vi "Firmware Filename Parser.vi"(0 "filename":string, 7 "firmware name":string, 11 "current versions":u8[](array[numeric])) -> (8 "update firmware":bool)   [LabVIEW 2010]
panel:
  out "assembly v (file)":dbl
  out "hw v (file)":dbl
  out "harp v (file)":dbl
  out "fw v (file)":dbl
  out "hw v (current)":dbl
  out "ass v (current)":dbl
  out "harp v (current)":dbl
  out "fw v (current)":dbl
  out "fw v":string
  out "harp v":string
  out "hw v":string
  out "assembly v":string
  out "assembly":string
  out "hw":string
  out "harp":string
  out "fw":string
  # "Delete this labels (debug only):"
  # "LedArray-fw2.2-harp1.4-hw1.x-ass0.hex"
  # "LedArray-fw2.2-harp1.4-hw1.3-ass0.hex"
  # "Behavior-fw2.2-harp1.4-hw1.0-ass2.hex"
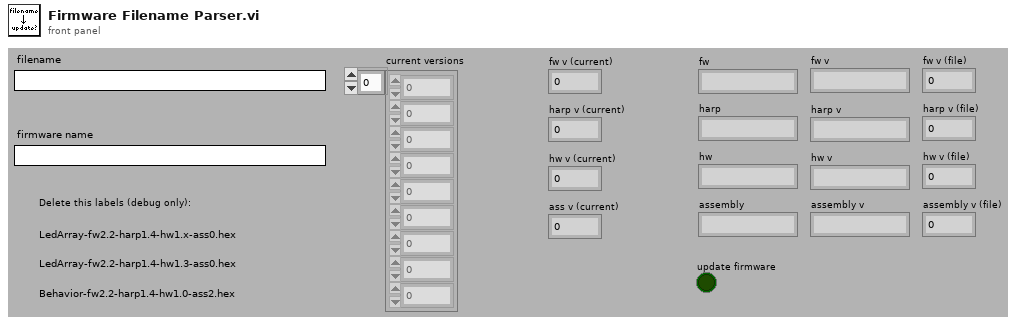
[diagram p1: front panel]
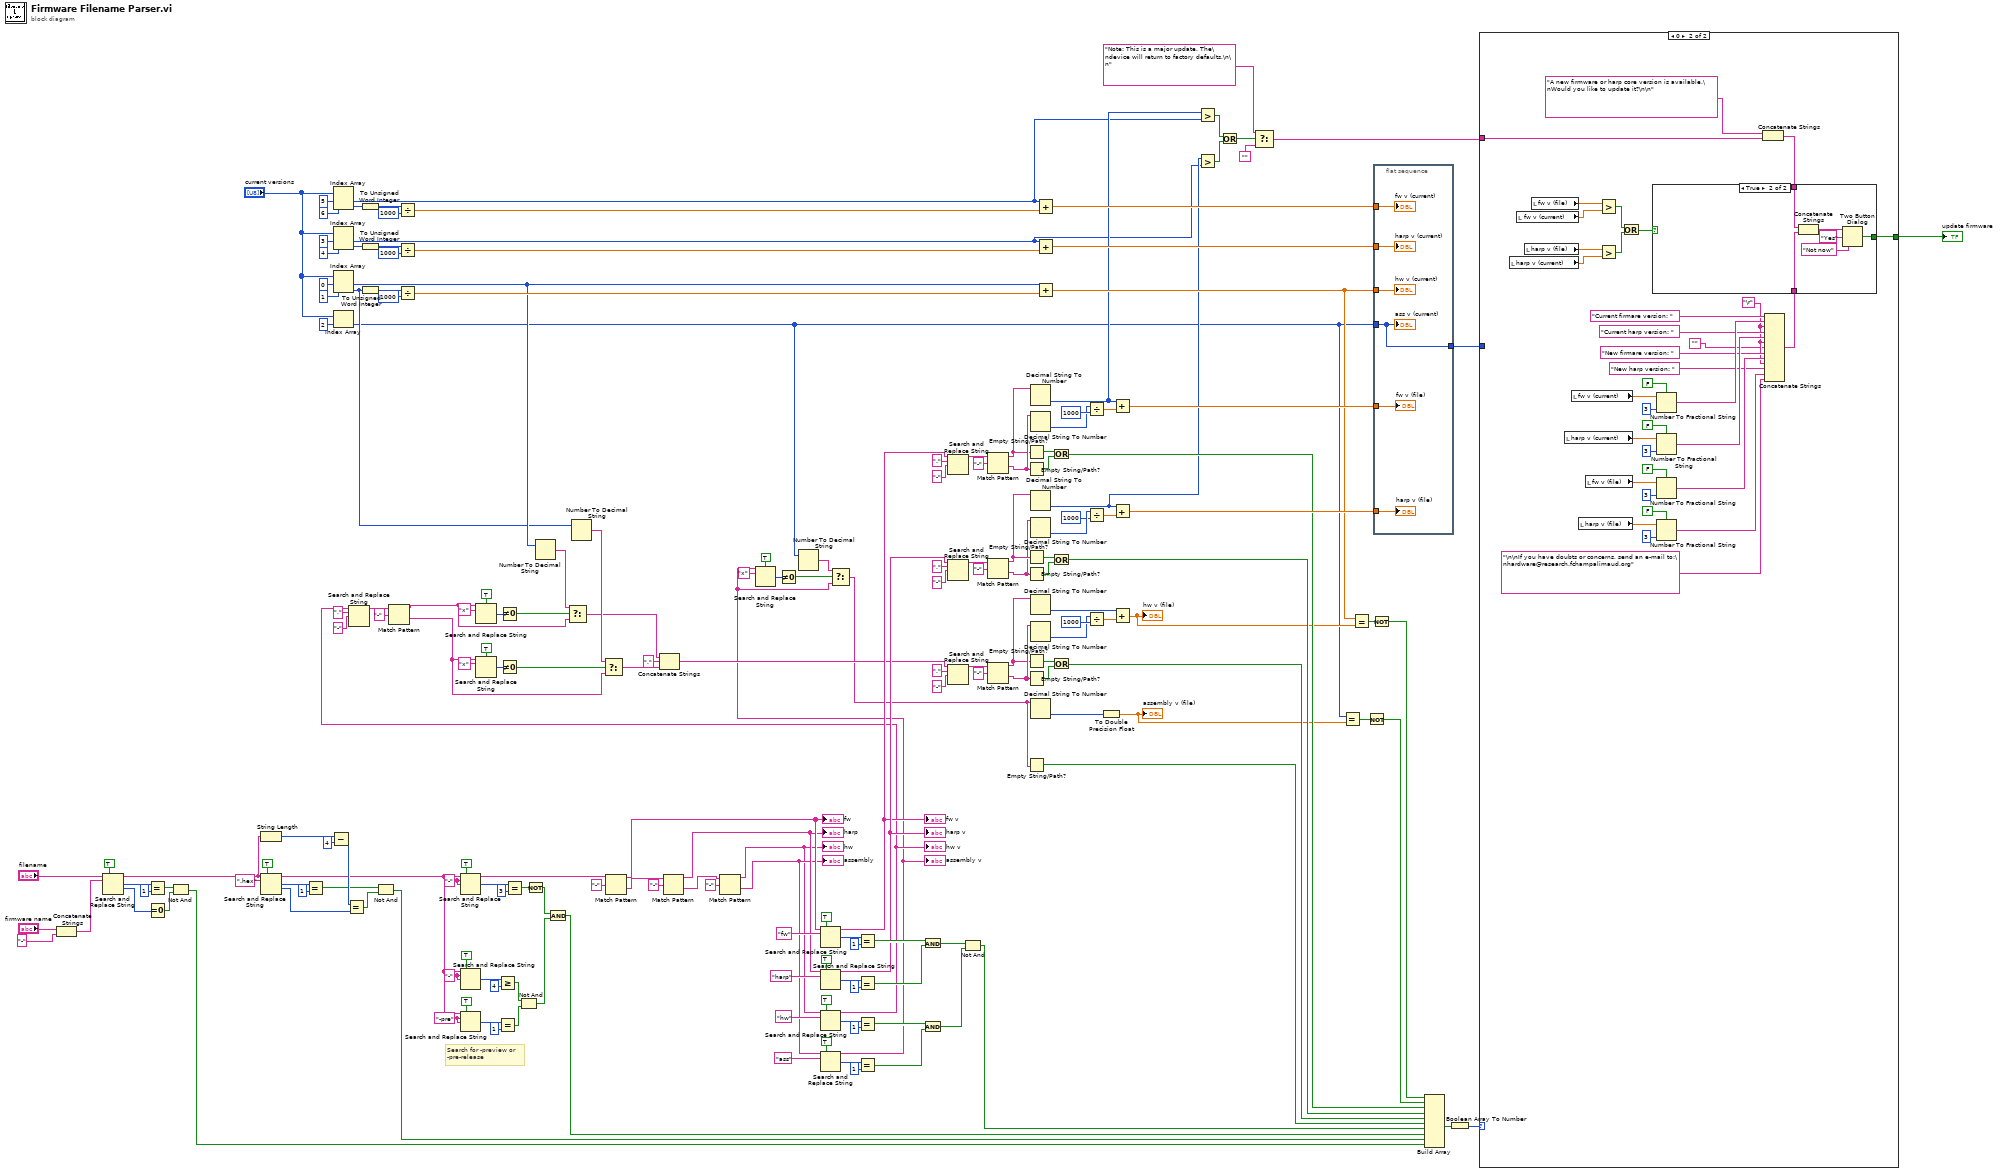
[diagram p0: block diagram]
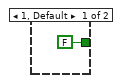
[diagram p2: hidden frame]
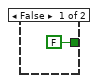
[diagram p3: hidden frame]
diagram:
  w7 = "-pre" ("search string")
  w12 = "-" ("search string")
  w170 = "-" ("search string")
  # "Search for -preview or\n-pre-release"
  n1 = Concatenate Strings("firmware name", "-" ("string")) -> (w188:string)
  n2 = Search and Replace String(replace all?=TRUE ("replace all? (F)"), input string="filename", search string=w188) -> (result string=w180:string, number of replacements=w187:i32, offset past replacement=w186:i32)  [unwired: 5 in, 1 out]
  n3 = Equal?(x=w187, y=1) -> (x = y?=w183:bool)
  n4 = Equal To 0?(x=w186) -> (x = 0?=w184:bool)
  n5 = Not And(1:w184, 2:w183) -> (0:w167:bool)
  n6 = String Length(string=w180) -> (length=w178:i32)
  n7 = Search and Replace String(replace all?=TRUE ("replace all? (F)"), input string=w180, search string=".hex") -> (result string=w5:string, number of replacements=w182:i32, offset past replacement=w175:i32)  [unwired: 5 in, 1 out]
  n8 = Equal?(x=w182, y=1) -> (x = y?=w173:bool)
  n9 = Subtract(x=w178, y=4) -> (x-y=w176:i32)
  n10 = Index Array(array="current versions", index #1=5 ("index"), index #2=6 ("index")) -> (element #1=w52:u8, element #2=w129:u8)
  n11 = Index Array(array="current versions", index #1=3 ("index"), index #2=4 ("index")) -> (element #1=w50:u8, element #2=w120:u8)
  n12 = Index Array(array="current versions", index #1=0 ("index"), index #2=1 ("index")) -> (element #1=w37:u8, element #2=w34:u8)
  n13 = Index Array(array="current versions", index=2) -> (element=w14:u8)
  n14 = Equal?(x=w176, y=w175) -> (x = y?=w174:bool)
  n15 = To Unsigned Word Integer(number=w129) -> (unsigned 16bit integer=w127:u16)
  n16 = To Unsigned Word Integer(number=w120) -> (unsigned 16bit integer=w122:u16)
  n17 = To Unsigned Word Integer(number=w34) -> (unsigned 16bit integer=w115:u16)
  n18 = Not And(1:w174, 2:w173) -> (0:w168:bool)
  n19 = Divide(x=w127, y=u16 1000) -> (x/y=w126:dbl)
  n20 = Divide(x=w122, y=u16 1000) -> (x/y=w123:dbl)
  n21 = Divide(x=w115, y=u16 1000) -> (x/y=w116:dbl)
  n22 = Search and Replace String(replace all?=TRUE ("replace all? (F)"), input string=w5, search string=w170, replace string=w170) -> (result string=w163:string, number of replacements=w171:i32)  [unwired: 4 in, 2 out]
  n23 = Search and Replace String(replace all?=TRUE ("replace all? (F)"), input string=w5, search string=w12, replace string=w12) -> (number of replacements=w11:i32)  [unwired: 4 in, 3 out]
  n24 = Search and Replace String(replace all?=TRUE ("replace all? (F)"), input string=w5, search string=w7, replace string=w7) -> (number of replacements=w8:i32)  [unwired: 4 in, 3 out]
  n25 = Greater Or Equal?(x=w11, y=4) -> (x >= y?=w3:bool)
  n26 = Equal?(x=w8, y=1) -> (x = y?=w4:bool)
  n27 = Equal?(x=w171, y=3) -> (x = y?=w169:bool)
  n28 = Not And(1:w4, 2:w3) -> (0:w1:bool)
  n29 = Not(x=w169) -> (.not. x?=w105:bool)
  n30 = Number To Decimal String(number=w37) -> (decimal integer string=w36:string)  [unwired: 1 in]
  n31 = And(x=w105, y=w1) -> (x .and. y?=w2:bool)
  n32 = Number To Decimal String(number=w34) -> (decimal integer string=w35:string)  [unwired: 1 in]
  n33 = Match Pattern(string=w163, regular expression="-") -> (before substring=w141:string, after substring=w160:string)  [unwired: 1 in, 2 out]
  "fw" <- w141
  n34 = Match Pattern(string=w160, regular expression="-") -> (before substring=w140:string, after substring=w158:string)  [unwired: 1 in, 2 out]
  "harp" <- w140
  n35 = Match Pattern(string=w158, regular expression="-") -> (before substring=w39:string, after substring=w139:string)  [unwired: 1 in, 2 out]
  "hw" <- w39
  "assembly" <- w139
  n36 = Number To Decimal String(number=w14) -> (decimal integer string=w17:string)  [unwired: 1 in]
  n37 = Search and Replace String(replace all?=TRUE ("replace all? (F)"), input string=w141, search string="fw") -> (result string=w72:string, number of replacements=w155:i32)  [unwired: 5 in, 2 out]
  "fw v" <- w72
  n38 = Search and Replace String(replace all?=TRUE ("replace all? (F)"), input string=w140, search string="harp") -> (result string=w73:string, number of replacements=w152:i32)  [unwired: 5 in, 2 out]
  "harp v" <- w73
  n39 = Search and Replace String(replace all?=TRUE ("replace all? (F)"), input string=w39, search string="hw") -> (result string=w26:string, number of replacements=w147:i32)  [unwired: 5 in, 2 out]
  "hw v" <- w26
  n40 = Search and Replace String(input string=w26, search string=".", replace string="-" ("replace string (\"\")")) -> (result string=w25:string)  [unwired: 5 in, 3 out]
  n41 = Match Pattern(string=w25, regular expression="-") -> (before substring=w24:string, after substring=w23:string)  [unwired: 1 in, 2 out]
  n42 = Search and Replace String(case sensitive?=TRUE ("ignore case? (F)"), input string=w24, search string="x") -> (number of replacements=w43:i32)  [unwired: 5 in, 3 out]
  n43 = Search and Replace String(case sensitive?=TRUE ("ignore case? (F)"), input string=w23, search string="x") -> (number of replacements=w42:i32)  [unwired: 5 in, 3 out]
  n44 = Not Equal To 0?(x=w43) -> (x != 0?=w38:bool)
  n45 = Not Equal To 0?(x=w42) -> (x != 0?=w30:bool)
  n46 = Select(t=w36, s=w38, f=w24) -> (s? t:f=w33:string)
  n47 = Select(t=w35, s=w30, f=w23) -> (s? t:f=w32:string)
  n48 = Concatenate Strings(w33, "." ("string"), w32) -> (w22:string)
  n49 = Search and Replace String(replace all?=TRUE ("replace all? (F)"), input string=w139, search string="ass") -> (result string=w16:string, number of replacements=w144:i32)  [unwired: 5 in, 2 out]
  "assembly v" <- w16
  n50 = Search and Replace String(case sensitive?=TRUE ("ignore case? (F)"), input string=w16, search string="x") -> (number of replacements=w19:i32)  [unwired: 5 in, 3 out]
  n51 = Not Equal To 0?(x=w19) -> (x != 0?=w18:bool)
  n52 = Select(t=w17, s=w18, f=w16) -> (s? t:f=w15:string)
  n53 = Equal?(x=w155, y=1) -> (x = y?=w138:bool)
  n54 = Equal?(x=w152, y=1) -> (x = y?=w137:bool)
  n55 = Equal?(x=w147, y=1) -> (x = y?=w136:bool)
  n56 = Equal?(x=w144, y=1) -> (x = y?=w135:bool)
  n57 = And(x=w138, y=w137) -> (x .and. y?=w134:bool)
  n58 = And(x=w136, y=w135) -> (x .and. y?=w133:bool)
  n59 = Search and Replace String(input string=w72, search string=".", replace string="-" ("replace string (\"\")")) -> (result string=w100:string)  [unwired: 5 in, 3 out]
  n60 = Search and Replace String(input string=w73, search string=".", replace string="-" ("replace string (\"\")")) -> (result string=w95:string)  [unwired: 5 in, 3 out]
  n61 = Search and Replace String(input string=w22, search string=".", replace string="-" ("replace string (\"\")")) -> (result string=w76:string)  [unwired: 5 in, 3 out]
  n62 = Not And(1:w133, 2:w134) -> (0:w132:bool)
  n63 = Match Pattern(string=w100, regular expression="-") -> (before substring=w106:string, after substring=w107:string)  [unwired: 1 in, 2 out]
  n64 = Match Pattern(string=w95, regular expression="-") -> (before substring=w90:string, after substring=w89:string)  [unwired: 1 in, 2 out]
  n65 = Match Pattern(string=w76, regular expression="-") -> (before substring=w81:string, after substring=w82:string)  [unwired: 1 in, 2 out]
  n66 = Empty String/Path?(string/path=w106) -> (empty?=w108:bool)
  n67 = Empty String/Path?(string/path=w107) -> (empty?=w109:bool)
  n68 = Empty String/Path?(string/path=w90) -> (empty?=w88:bool)
  n69 = Empty String/Path?(string/path=w89) -> (empty?=w87:bool)
  n70 = Empty String/Path?(string/path=w81) -> (empty?=w83:bool)
  n71 = Empty String/Path?(string/path=w82) -> (empty?=w84:bool)
  n72 = Empty String/Path?(string/path=w15) -> (empty?=w68:bool)
  n73 = Decimal String To Number(string=w106) -> (number=w53:i32)  [unwired: 2 in, 1 out]
  n74 = Decimal String To Number(string=w107) -> (number=w101:i32)  [unwired: 2 in, 1 out]
  n75 = Decimal String To Number(string=w90) -> (number=w51:i32)  [unwired: 2 in, 1 out]
  n76 = Decimal String To Number(string=w89) -> (number=w94:i32)  [unwired: 2 in, 1 out]
  n77 = Decimal String To Number(string=w81) -> (number=w78:i32)  [unwired: 2 in, 1 out]
  n78 = Decimal String To Number(string=w82) -> (number=w77:i32)  [unwired: 2 in, 1 out]
  n79 = Decimal String To Number(string=w15) -> (number=w66:i32)  [unwired: 2 in, 1 out]
  n80 = Add(x=w52, y=w126) -> (x+y=w125:dbl)
  n81 = Add(x=w50, y=w123) -> (x+y=w124:dbl)
  n82 = Add(x=w37, y=w116) -> (x+y=w63:dbl)
  n83 = Or(x=w108, y=w109) -> (x .or. y?=w71:bool)
  n84 = Or(x=w88, y=w87) -> (x .or. y?=w70:bool)
  n85 = Or(x=w83, y=w84) -> (x .or. y?=w69:bool)
  n86 = Divide(x=w101, y=u16 1000) -> (x/y=w103:dbl)
  n87 = Divide(x=w94, y=u16 1000) -> (x/y=w92:dbl)
  n88 = Divide(x=w77, y=u16 1000) -> (x/y=w79:dbl)
  n89 = To Double Precision Float(number=w66) -> (double precision float=w65:dbl)
  "assembly v (file)" <- w65
  n90 = Add(x=w53, y=w103) -> (x+y=w102:dbl)
  n91 = Add(x=w51, y=w92) -> (x+y=w93:dbl)
  n92 = Add(x=w78, y=w79) -> (x+y=w64:dbl)
  "hw v (file)" <- w64
  n93 = Greater?(x=w53, y=w52) -> (0:w55:bool)
  n94 = Greater?(x=w51, y=w50) -> (0:w54:bool)
  n95 = Or(x=w55, y=w54) -> (x .or. y?=w49:bool)
  n96 = Select(t="Note: This is a major update. The\ndevice will return to factory defaults.\n\n" ("message"), s=w49, f="") -> (s? t:f=w46:string)
  n97 = Equal?(x=w14, y=w65) -> (x = y?=w61:bool)
  n98 = Equal?(x=w63, y=w64) -> (x = y?=w62:bool)
  n99 = Not(x=w61) -> (.not. x?=w60:bool)
  n100 = Not(x=w62) -> (.not. x?=w59:bool)
  n101 = flat-sequence {
    tunnel: w125 -> [w197]
    tunnel: w124 -> [w196]
    tunnel: w102 -> [w195]
    tunnel: w93 -> [w194]
    tunnel: w14 -> [w192]
    tunnel: w63 -> [w193]
    tunnel: [w192] -> w57
    frame #0 {
      "fw v (current)" <- w197
      "harp v (current)" <- w196
      "hw v (current)" <- w193
      "ass v (current)" <- w192
      "fw v (file)" <- w195
      "harp v (file)" <- w194
    }
  }
  n102 = Build Array(w59, w60, w71, w70, w69, w68, w132, w2, w168, w167) -> (w67:bool[])
  n103 = Boolean Array To Number(Boolean array=w67) -> (number=w58:u32)
  n104 = case shown="0" w58 {
    tunnel: w57 -> [_ _]
    tunnel: [FALSE ("T button?") w206] -> w56
    tunnel: w46 -> [_ w202]
    frame 1, Default {
    }
    frame 0 {
      w211 = "\r"
      n105 = local read "harp v (current)"() -> (w231:dbl)
      n106 = local read "fw v (current)"() -> (w232:dbl)
      n107 = local read "harp v (file)"() -> (w230:dbl)
      n108 = local read "fw v (file)"() -> (w233:dbl)
      n109 = local read "harp v (current)"() -> (w222:dbl)
      n110 = local read "fw v (current)"() -> (w225:dbl)
      n111 = local read "harp v (file)"() -> (w221:dbl)
      n112 = local read "fw v (file)"() -> (w218:dbl)
      n113 = Greater?(x=w233, y=w232) -> (0:w228:bool)
      n114 = Greater?(x=w230, y=w231) -> (0:w229:bool)
      n115 = Or(x=w228, y=w229) -> (x .or. y?=w207:bool)
      n116 = Number To Fractional String(use system decimal point (T)=FALSE, number=w225, precision (6)=i16 3) -> (F-format string=w216:string)  [unwired: 1 in]
      n117 = Number To Fractional String(use system decimal point (T)=FALSE, number=w222, precision (6)=i16 3) -> (F-format string=w214:string)  [unwired: 1 in]
      n118 = Number To Fractional String(use system decimal point (T)=FALSE, number=w218, precision (6)=i16 3) -> (F-format string=w212:string)  [unwired: 1 in]
      n119 = Number To Fractional String(use system decimal point (T)=FALSE, number=w221, precision (6)=i16 3) -> (F-format string=w209:string)  [unwired: 1 in]
      n120 = Concatenate Strings("A new firmware or harp core version is available.\nWould you like to update it?\n\n" ("message"), w202) -> (w200:string)
      n121 = Concatenate Strings("Current firmare version: " ("message"), w216, w211, "Current harp version: " ("message"), w214, w211, "", "New firmare version: " ("message"), w212, w211, "New harp version: " ("message"), w209, "\n\nIf you have doubts or concerns, send an e-mail to:\nhardware@research.fchampalimaud.org" ("message")) -> (w208:string)
      n122 = case shown="True" w207 {
        tunnel: w208 -> [_ w240]
        tunnel: [FALSE ("T button?") w236] -> w206
        tunnel: w200 -> [_ w235]
        frame False {
        }
        frame True {
          n123 = Concatenate Strings(w235, w240) -> (w239:string)
          n124 = Two Button Dialog(message=w239, 1:"Not now" ("F button name (\"Cancel\")"), 2:"Yes" ("T button name (\"OK\")")) -> (T button?=w236:bool)
        }
      }
    }
  }
  "update firmware" <- w56
